vi "Static Read.vi"(8 "error in (no error)":errorcluster, 11 "Abs_Complex Single Float in":refnum<class "Abs_Complex Single Float.lvclass">) -> (0 "error out":errorcluster, 2 "Value":csg, 3 "Abs_Complex Single Float out":refnum<class "Abs_Complex Single Float.lvclass">)   [LabVIEW 2021, in "Abs_Complex Single Float.lvclass"]
uses:
  Abs_Complex Single Float.lvclass
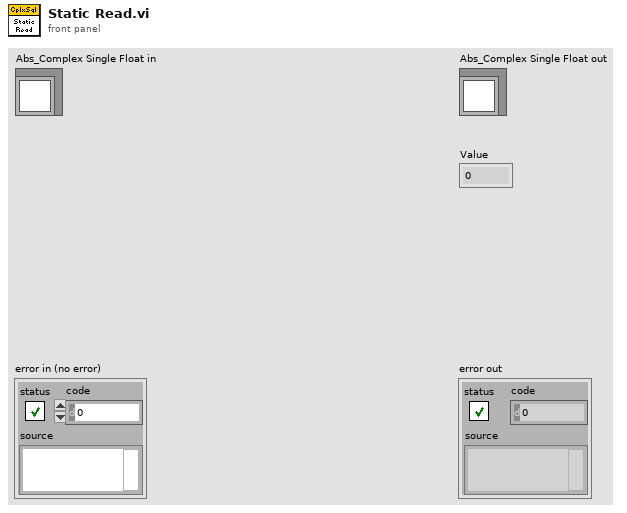
[diagram p1: front panel]
types:
  T1 = typedef "Abs_Complex Single Float.lvclass/Type.ctl" = csg
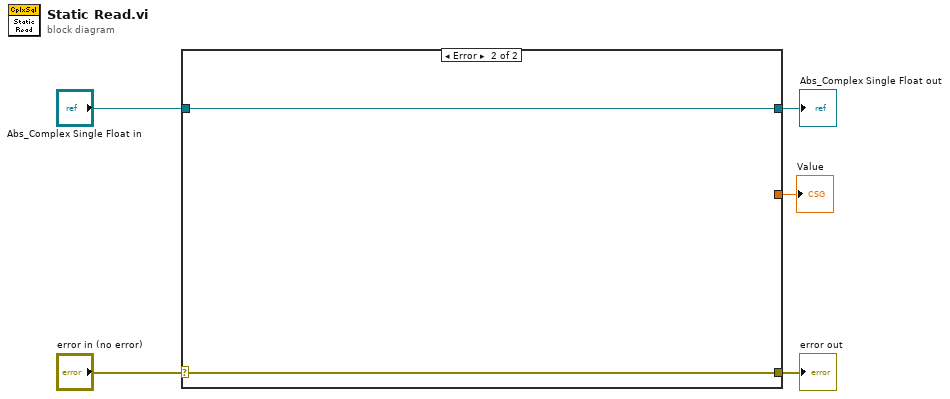
[diagram p0: block diagram]
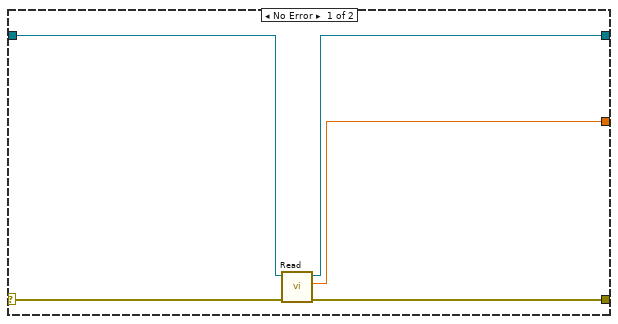
[diagram p2: hidden frame]
diagram:
  n1 = case shown="Error" "error in (no error)" {
    selector: "error in (no error)" -> [w10 w12]
    tunnel: [w9 w12] -> w4
    tunnel: [w7 w11] -> w2
    tunnel: "Abs_Complex Single Float in" -> [w8 w11]
    tunnel: [w6 _] -> w1
    frame No Error {
      n2 = call-dynamic "Read.vi"("error in (no error)"=w10, "Double Float.lvclass_340760 in"=w8) -> ("error out"=w9:errorcluster, "Value"=w6:T1, "Double Float.lvclass_340760 out"=w7:refnum<class "Abs_Complex Single Float.lvclass">)  [unwired: 7 in]
    }
    frame Error {
    }
  }
  "error out" <- w4
  "Abs_Complex Single Float out" <- w2
  "Value" <- w1
